vi "TRTDM Configure Range and Terminal Settings.vi"(0 "DAQmx Task In":refnum<k21>, 5 "Range and Terminal Settings":T1={"Global Settings"={"Min Temp (deg C)"=100.0, "Max Temp (deg C)"=0.0, "RTD Type"=12481, "Sensor Resistance \nat 0 deg C (Ohm)"=0.0001, "Resistance \nConfiguration"=3, "Current Excitation\nSource"=10200, "Current \nExcitation (A)"=0.001, "ADC Timing Mode"=16097}, "Specific Channel Settings"=[]} {"Specific Channel Settings"."Current Excitation Source" items=["Internal"=10200, "External"=10167]; "Specific Channel Settings"."Current Excitation (A)" format="%#.6p"; "Specific Channel Settings"."Resistance Configuration" items=["3-Wire"=3, "4-Wire"=4]; "Specific Channel Settings"."Sensor Resistance at 0 deg C (Ohm)" format="%1.2f"; "Specific Channel Settings"."RTD Type" items=["Pt3750"=12481, "Pt3851"=10071, "Pt3911"=12482, "Pt3916"=10069, "Pt3920"=10053, "Pt3928"=12483]; "Global Settings"."ADC Timing Mode" items=["Automatic"=16097, "High Resolution"=10195, "High Speed"=14712]; "Global Settings"."Sensor Resistance \nat 0 deg C (Ohm)" format="%.2f"; "Global Settings"."RTD Type" items=["Pt3750"=12481, "Pt3851"=10071, "Pt3911"=12482, "Pt3916"=10069, "Pt3920"=10053, "Pt3928"=12483]; "Global Settings"."Current Excitation\nSource" items=["Internal"=10200, "External"=10167]; "Global Settings"."Current \nExcitation (A)" format="%#.6p"; "Global Settings"."Resistance \nConfiguration" items=["3-Wire"=3, "4-Wire"=4]; "Global Settings"."Min Temp (deg C)" format="%.2f"; "Global Settings"."Max Temp (deg C)" format="%.2f"}, 11 "error in (no error)":errorcluster) -> (4 "DAQmx Task Out":refnum<k21>, 15 "error out":errorcluster)   [LabVIEW 2021, in "DAQ_Temperature RTD Measurement.lvlib"]
doc: "Configures the <B>Global and Specific</B> channels settings to the equivalent channels in DAQmx Task"
uses:
  DAQ_Temperature RTD Measurement.lvlib
  <resource>/objmgr/daqmx.rc
  Typedefs/Range and Terminal Settings.ctl
  Typedefs/Specific Channel Settings.ctl
  Typedefs/ADC Timing Mode.ctl
panel:
  # "Sensor Resistance at 0 deg C (Ohm)"
  # "Resistance Configuration"
  # "Current Excitation Source"
  # "Current Excitation (A)"
  # "Physical Channel Name"
  # "RTD Type"
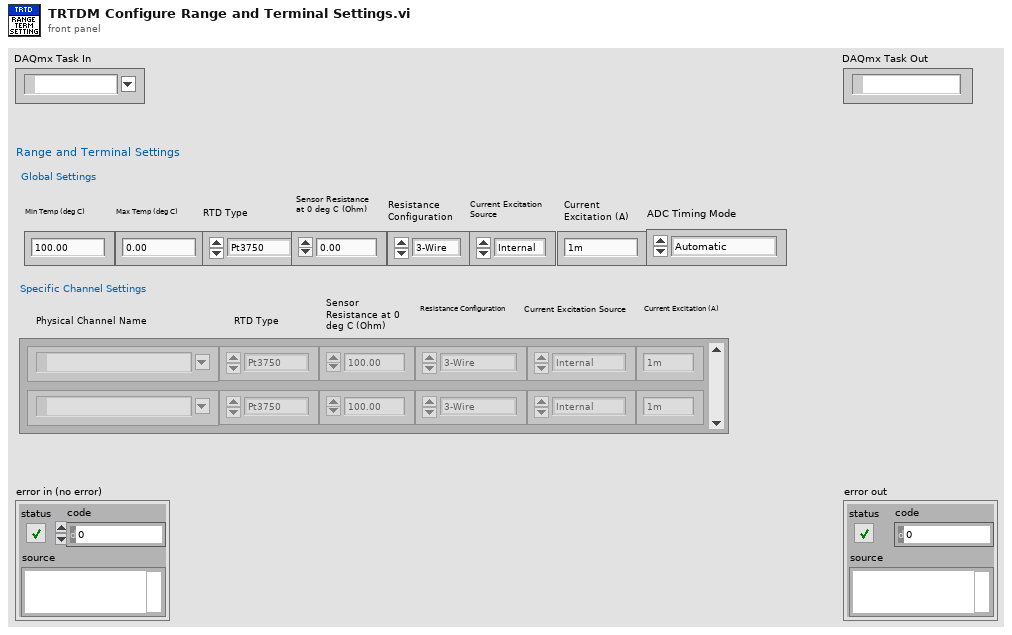
[diagram p1: front panel]
types:
  T1 = typedef "DAQ_Temperature RTD Measurement.lvlib/Range and Terminal Settings.ctl" = cluster{"Global Settings":cluster{"Min Temp (deg C)":dbl, "Max Temp (deg C)":dbl, "RTD Type":i32, "Sensor Resistance \nat 0 deg C (Ohm)":dbl, "Resistance \nConfiguration":i32, "Current Excitation\nSource":i32, "Current \nExcitation (A)":dbl, "ADC Timing Mode":T2}, "Specific Channel Settings":T3[]}
  T2 = typedef "DAQ_Temperature RTD Measurement.lvlib/ADC Timing Mode.ctl" = i32
  T3 = typedef "DAQ_Temperature RTD Measurement.lvlib/Specific Channel Settings.ctl" = cluster{"Active Channels":tag, "RTD Type":i32, "Sensor Resistance at 0 deg C (Ohm)":dbl, "Resistance Configuration":i32, "Current Excitation Source":i32, "Current Excitation (A)":dbl}
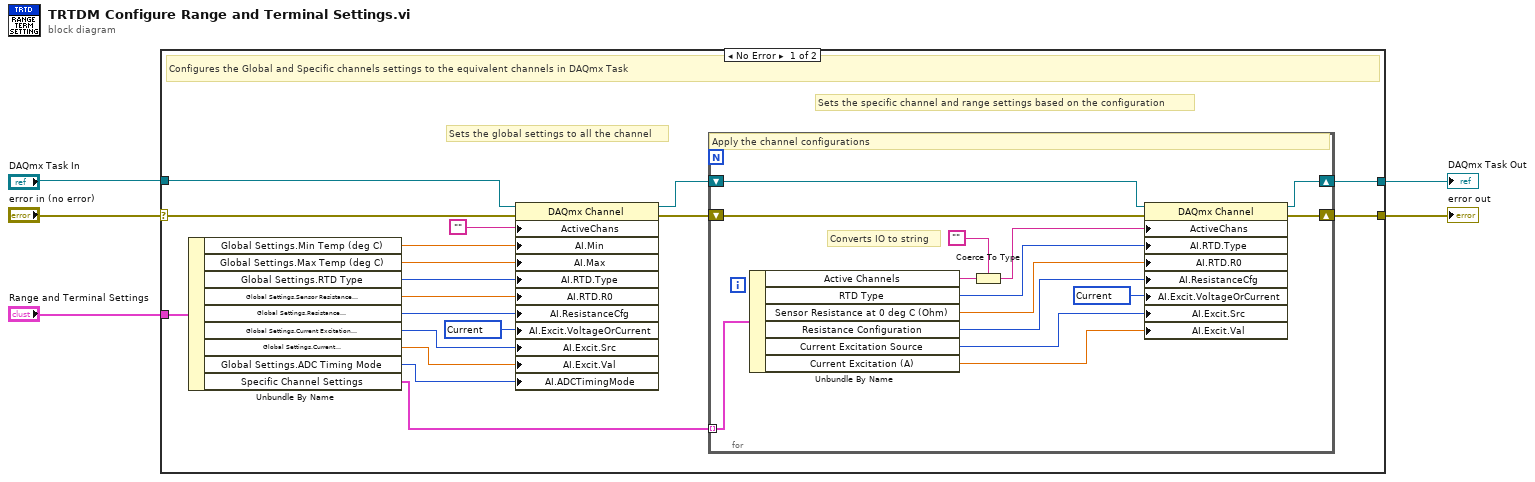
[diagram p0: block diagram]
diagram:
  n1 = case shown="No Error" "error in (no error)" {
    selector: "error in (no error)" -> [w17 w39]
    tunnel: "DAQmx Task In" -> [w19 w38]
    tunnel: "Range and Terminal Settings" -> [w16 _]
    tunnel: [w15 w38] -> w3
    tunnel: [w14 w39] -> w2
    frame No Error {
      w12 = 10134 items=["Voltage"=10322, "Current"=10134] ("AI.Excit.VoltageOrCurrent")
      # "Sets the specific channel and range settings based on the configuration"
      # "Sets the global settings to all the channel"
      # "Configures the Global and Specific channels settings to the equivalent channels in DAQmx Task"
      n2 = Unbundle By Name(w16) -> ("Global Settings.Min Temp (deg C)"=w22:dbl, "Global Settings.Max Temp (deg C)"=w23:dbl, "Global Settings.RTD Type"=w11:i32, "Global Settings.Sensor Resistance \nat 0 deg C (Ohm)"=w13:dbl, "Global Settings.Resistance \nConfiguration"=w10:i32, "Global Settings.Current Excitation\nSource"=w9:i32, "Global Settings.Current \nExcitation (A)"=w8:dbl, "Global Settings.ADC Timing Mode"=w6:T2, "Specific Channel Settings"=w7:T3[])
      n3 = property class="DAQmx Channel"(reference=w19, error in=w17, "ActiveChans"="", "AI.Min"=w22, "AI.Max"=w23, "AI.RTD.Type"=w11, "AI.RTD.R0"=w13, "AI.ResistanceCfg"=w10, "AI.Excit.VoltageOrCurrent"=w12, "AI.Excit.Src"=w9, "AI.Excit.Val"=w8, "AI.ADCTimingMode"=w6) -> (reference out=w20:refnum<k21>, error out=w18:errorcluster)
      n4 = for {
        shift-right: [w31] -> w15
        shift-left: w20 -> [w32]
        shift-right: [w30] -> w14
        shift-left: w18 -> [w33]
        tunnel: w7 -> [w37] mode=indexing
        w34 = 10134 items=["Voltage"=10322, "Current"=10134] ("AI.Excit.VoltageOrCurrent")
        # "Converts IO to string"
        # "Apply the channel configurations"
        n5 = Unbundle By Name(w37) -> ("Active Channels"=w35:tag, "RTD Type"=w28:i32, "Sensor Resistance at 0 deg C (Ohm)"=w27:dbl, "Resistance Configuration"=w26:i32, "Current Excitation Source"=w25:i32, "Current Excitation (A)"=w24:dbl)
        n6 = Coerce To Type(0:w35, 1:"") -> (2:w29:string)
        n7 = property class="DAQmx Channel"(reference=w32, error in=w33, "ActiveChans"=w29, "AI.RTD.Type"=w28, "AI.RTD.R0"=w27, "AI.ResistanceCfg"=w26, "AI.Excit.VoltageOrCurrent"=w34, "AI.Excit.Src"=w25, "AI.Excit.Val"=w24) -> (reference out=w31:refnum<k21>, error out=w30:errorcluster)
      }
    }
    frame Error {
      # "Error case - Do nothing"
    }
  }
  "DAQmx Task Out" <- w3
  "error out" <- w2
